vi "Variant Is Empty Object.vi"(1 "Variant":variant) -> (0 "Is Empty Object?":bool)   [LabVIEW 2018, in "labview_json.lvlib"]
uses:
  labview_json.lvlib
  <vilib>/Utility/Data Type/Type Definitions/Data Type.ctl
  <vilib>/Utility/Data Type/NI_Data Type.lvlib
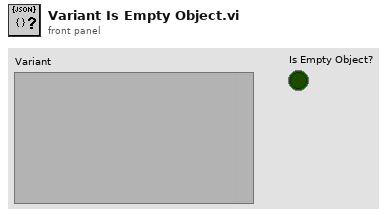
[diagram p1: front panel]
types:
  T1 = typedef "NI_Data Type.lvlib/Data Type.ctl" = enum8{"Invalid Type", "Void", "I8", "I16", "I32", "I64", "U8", "U16", "U32", "U64", "Single Float", "Double Float", "Extended Float", "Single Complex", "Double Complex", "Extended Complex", "Enum U8", "Enum U16", "Enum U32", "Enum U64", "Single Float With Unit", "Double Float With Unit", "Extended Float With Unit", "Single Complex with Unit", "Double Complex with Unit", "Extended Complex with Unit", "Boolean", "String", "Path", "Picture", "Tag", "Array", "Cluster", "Variant", "LV Variant", "Waveform", "Timestamp", "Digital Waveform", "Digital Data", "ExpressData", "Refnum", "External Data", "VI", "Poly VI", "LabVIEW Class Instance", "Fixed Point", "Set Collection", "Map Collection"}
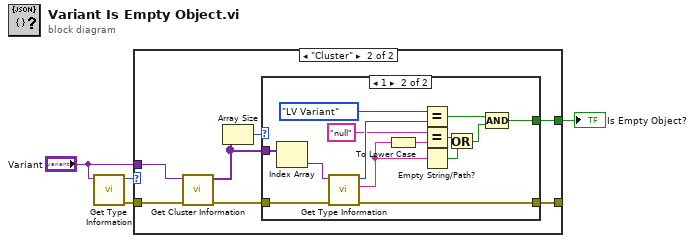
[diagram p0: block diagram]
diagram:
  n1 = call <vilib>:"Get Type Information.vi"("variant"="Variant") -> ("error out"=w4:errorcluster, "type"=w3:T1)  [unwired: 6 in, 3 out]
  n2 = case shown="\"Cluster\"" w3 {
    tunnel: "Variant" -> [_ w7]
    tunnel: [_ w11] -> w1
    tunnel: w4 -> [w5 w9]
    tunnel: [w5 w10] -> _
    frame Default {
    }
    frame "Cluster" {
      n3 = call <vilib>:"Get Cluster Information.vi"("error in (no error)"=w9, "variant"=w7) -> ("error out"=w8:errorcluster, "cluster elements"=w6:variant[])  [unwired: 8 in]
      n4 = Array Size(array=w6) -> (size(s)=w12:i32)
      n5 = case shown="1" w12 {
        tunnel: w6 -> [_ w27]
        tunnel: [_ w25] -> w11
        tunnel: w8 -> [w13 w24]
        tunnel: [w13 w20] -> w10
        frame Default {
        }
        frame 1 {
          n6 = Index Array(array=w27) -> (element=w23:variant)  [unwired: 1 in]
          n7 = call <vilib>:"Get Type Information.vi"("error in (no error)"=w24, "variant"=w23) -> ("error out"=w20:errorcluster, "name"=w17:string, "type"=w22:T1)  [unwired: 5 in, 2 out]
          n8 = To Lower Case(string=w17) -> (all lower case string=w14:string)
          n9 = Equal?(x=Data_Type."LV Variant" ("Type"), y=w22) -> (x = y?=w26:bool)
          n10 = Equal?(x="null", y=w14) -> (x = y?=w18:bool)
          n11 = Empty String/Path?(string/path=w17) -> (empty?=w15:bool)
          n12 = Or(x=w18, y=w15) -> (x .or. y?=w16:bool)
          n13 = Compound Arithmetic op=AND(w26, w16) -> (w25:bool)
        }
      }
    }
  }
  "Is Empty Object?" <- w1
